vi "Approximate Polygon (Convex-Hull).vi"(5 "Epsilon % (Default: -1 ignore)":dbl=-1.0 format="%#_13g", 7 "Ensure Convex? (Default: True)":bool=TRUE, 8 "error in (no error)":errorcluster, 10 "N-Sides":u8, 11 "Points in":T1[](array[typedef])) -> (0 "error out":errorcluster, 3 "Points out":T1[](array[typedef]))   [LabVIEW 2020, in "shape.lvlib"]
doc: "Approximates a polygon with a convex hull so that the difference between the contour area of the original contour and the new polygon is minimal.\n\nIt uses a greedy algorithm for contracting two vertices into one in such a way that the additional area is minimal. Straight lines formed by each edge of the convex contour are drawn and the areas of the resulting triangles are considered. Each vertex will lie either on the original contour or outside it."
uses:
  common/Image Point (Integer).ctl
  shape.lvlib
  common/common.lvlib
  common/bin/gartoolkit_32-1.dll
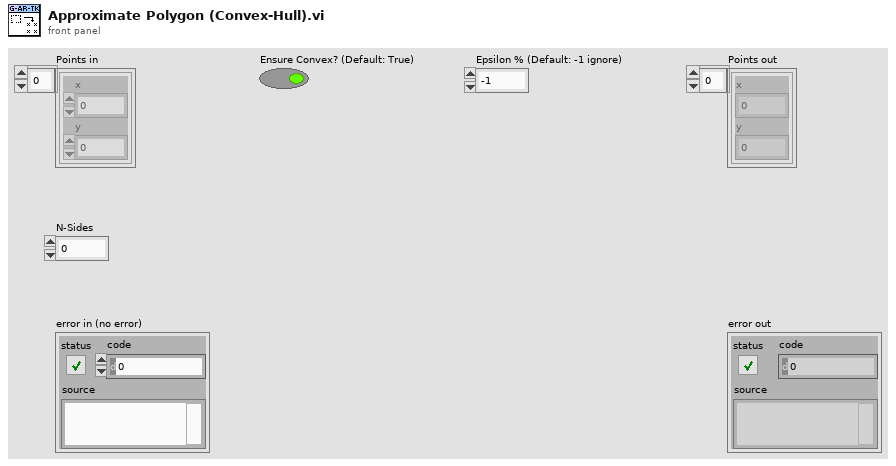
[diagram p1: front panel]
types:
  T1 = typedef "common.lvlib/Image Point (Integer).ctl" = cluster{"x":i32, "y":i32}
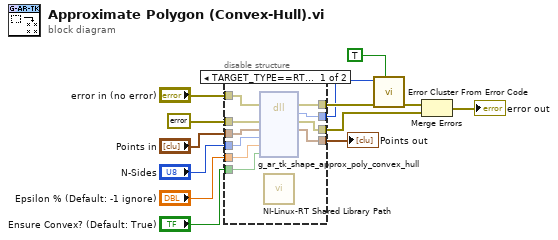
[diagram p0: block diagram]
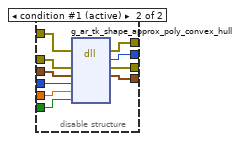
[diagram p2: hidden frame]
diagram:
  n1 = disable-structure shown="TARGET_TYPE==RT&&OS==Linux" {
    disable-tunnel: "error in (no error)" -> [w23 w33]
    disable-tunnel: errorcluster {"status"=FALSE, "code"=0, "source"=""} ("error constant") -> [w20 w32]
    disable-tunnel: "Points in" -> [w19 w31]
    disable-tunnel: "Epsilon % (Default: -1 ignore)" -> [w17 w30]
    disable-tunnel: "Ensure Convex? (Default: True)" -> [w16 w29]
    disable-tunnel: [w22 w28] -> w6
    disable-tunnel: [w21 w27] -> w5
    disable-tunnel: [w14 w26] -> w4
    disable-tunnel: [w15 w25] -> w3
    disable-tunnel: "N-Sides" -> [w18 w24]
    frame condition #0 {
      n2 = dll-call lib="?" fn="g_ar_tk_shape_approx_poly_convex_hull" ("g_ar_toolkit.*.*:g_ar_tk_image_draw_line")(error in=w23, "error_cluster"=w20, "points"=w19, "n_sides"=w18, "epsilon_pct"=w17, "ensure_convex"=w16) -> (error out=w22:errorcluster, "MgErr"=w21:i32, "error_cluster"=w14:errorcluster, "points"=w15:T1[])  [unwired: 5 in, 1 out]
      n3 = call "NI-Linux-RT Shared Library Path.vi"() -> ()  [unwired: 1 out]
    }
    frame condition #1 (active) {
      n4 = dll-call lib="C:/serenial/lib/g-augmented-reality-toolkit/LabVIEW/common/bin/gartoolkit_*-1.*" fn="g_ar_tk_shape_approx_poly_convex_hull" ("g_ar_toolkit.*.*:g_ar_tk_image_draw_line")(error in=w33, "error_cluster"=w32, "points"=w31, "n_sides"=w24, "epsilon_pct"=w30, "ensure_convex"=w29) -> (error out=w28:errorcluster, "MgErr"=w27:i32, "error_cluster"=w26:errorcluster, "points"=w25:T1[])  [unwired: 5 in, 1 out]
    }
  }
  "Points out" <- w3
  n5 = call <vilib>:"Error Cluster From Error Code.vi"("show call chain? (False)"=TRUE, "error in (no error)"=w6, "error code (0)"=w5) -> ("error out"=w12:errorcluster)  [unwired: 6 in]
  n6 = Merge Errors(w12, w4) -> (→"error out":errorcluster)
